vi "ID Finder.vi"(6 "cluster":T3 {"data[0]"."payload" format="%x"; "data[0]"."timestamp" format="%<%.7X\n%x>T"; "data[0]"."type" items=["CAN Data"=0, "CAN Remote"=1, "CAN Bus Error"=2, "CAN 2.0 Data"=8, "CAN FD Data"=16, "CAN FD+BRS Data"=24, "J1939 Data"=192, "Delay"=224, "Log Trigger"=225, "Start Trigger"=226]; "data[0]"."identifier" format="%x"; "data[1]"."payload" format="%x"; "data[1]"."timestamp" format="%<%.7X\n%x>T"; "data[1]"."type" items=["CAN Data"=0, "CAN Remote"=1, "CAN Bus Error"=2, "CAN 2.0 Data"=8, "CAN FD Data"=16, "CAN FD+BRS Data"=24, "J1939 Data"=192, "Delay"=224, "Log Trigger"=225, "Start Trigger"=226]; "data[1]"."identifier" format="%x"; "data[2]"."payload" format="%x"; "data[2]"."timestamp" format="%<%.7X\n%x>T"; "data[2]"."type" items=["CAN Data"=0, "CAN Remote"=1, "CAN Bus Error"=2, "CAN 2.0 Data"=8, "CAN FD Data"=16, "CAN FD+BRS Data"=24, "J1939 Data"=192, "Delay"=224, "Log Trigger"=225, "Start Trigger"=226]; "data[2]"."identifier" format="%x"; "data[3]"."payload" format="%x"; "data[3]"."timestamp" format="%<%.7X\n%x>T"; "data[3]"."type" items=["CAN Data"=0, "CAN Remote"=1, "CAN Bus Error"=2, "CAN 2.0 Data"=8, "CAN FD Data"=16, "CAN FD+BRS Data"=24, "J1939 Data"=192, "Delay"=224, "Log Trigger"=225, "Start Trigger"=226]; "data[3]"."identifier" format="%x"; "data[4]"."payload" format="%x"; "data[4]"."timestamp" format="%<%.7X\n%x>T"; "data[4]"."type" items=["CAN Data"=0, "CAN Remote"=1, "CAN Bus Error"=2, "CAN 2.0 Data"=8, "CAN FD Data"=16, "CAN FD+BRS Data"=24, "J1939 Data"=192, "Delay"=224, "Log Trigger"=225, "Start Trigger"=226]; "data[4]"."identifier" format="%x"; "data[5]"."payload" format="%x"; "data[5]"."timestamp" format="%<%.7X\n%x>T"; "data[5]"."type" items=["CAN Data"=0, "CAN Remote"=1, "CAN Bus Error"=2, "CAN 2.0 Data"=8, "CAN FD Data"=16, "CAN FD+BRS Data"=24, "J1939 Data"=192, "Delay"=224, "Log Trigger"=225, "Start Trigger"=226]; "data[5]"."identifier" format="%x"; "data[6]"."payload" format="%x"; "data[6]"."timestamp" format="%<%.7X\n%x>T"; "data[6]"."type" items=["CAN Data"=0, "CAN Remote"=1, "CAN Bus Error"=2, "CAN 2.0 Data"=8, "CAN FD Data"=16, "CAN FD+BRS Data"=24, "J1939 Data"=192, "Delay"=224, "Log Trigger"=225, "Start Trigger"=226]; "data[6]"."identifier" format="%x"; "data[7]"."payload" format="%x"; "data[7]"."timestamp" format="%<%.7X\n%x>T"; "data[7]"."type" items=["CAN Data"=0, "CAN Remote"=1, "CAN Bus Error"=2, "CAN 2.0 Data"=8, "CAN FD Data"=16, "CAN FD+BRS Data"=24, "J1939 Data"=192, "Delay"=224, "Log Trigger"=225, "Start Trigger"=226]; "data[7]"."identifier" format="%x"; "data[8]"."payload" format="%x"; "data[8]"."timestamp" format="%<%.7X\n%x>T"; "data[8]"."type" items=["CAN Data"=0, "CAN Remote"=1, "CAN Bus Error"=2, "CAN 2.0 Data"=8, "CAN FD Data"=16, "CAN FD+BRS Data"=24, "J1939 Data"=192, "Delay"=224, "Log Trigger"=225, "Start Trigger"=226]; "data[8]"."identifier" format="%x"}) -> (0 "Data Type":T1 items=["CAN Data"=0, "CAN Remote"=1, "CAN Bus Error"=2, "CAN 2.0 Data"=8, "CAN FD Data"=16, "CAN FD+BRS Data"=24, "J1939 Data"=192, "Delay"=224, "Log Trigger"=225, "Start Trigger"=226], 1 "ID STRING":string, 2 "Payload":u8[](array[numeric]), 3 "Timestamp":timestamp, 4 "Identifier":u32)   [LabVIEW 2022 SP3]
uses:
  <vilib>/xnet/xnet.llb/XNET Frame CAN.ctl
  <vilib>/xnet/xnet.llb/XNET Frame Type CAN.ctl
  C:/Users/k90011005/Desktop/Practicas/C#/String-Hexa/bin/Debug/String-Hexa.dll
  Users/k90011005/Desktop/Practicas/C#/String-Hexa/bin/Debug/String-Hexa.dll
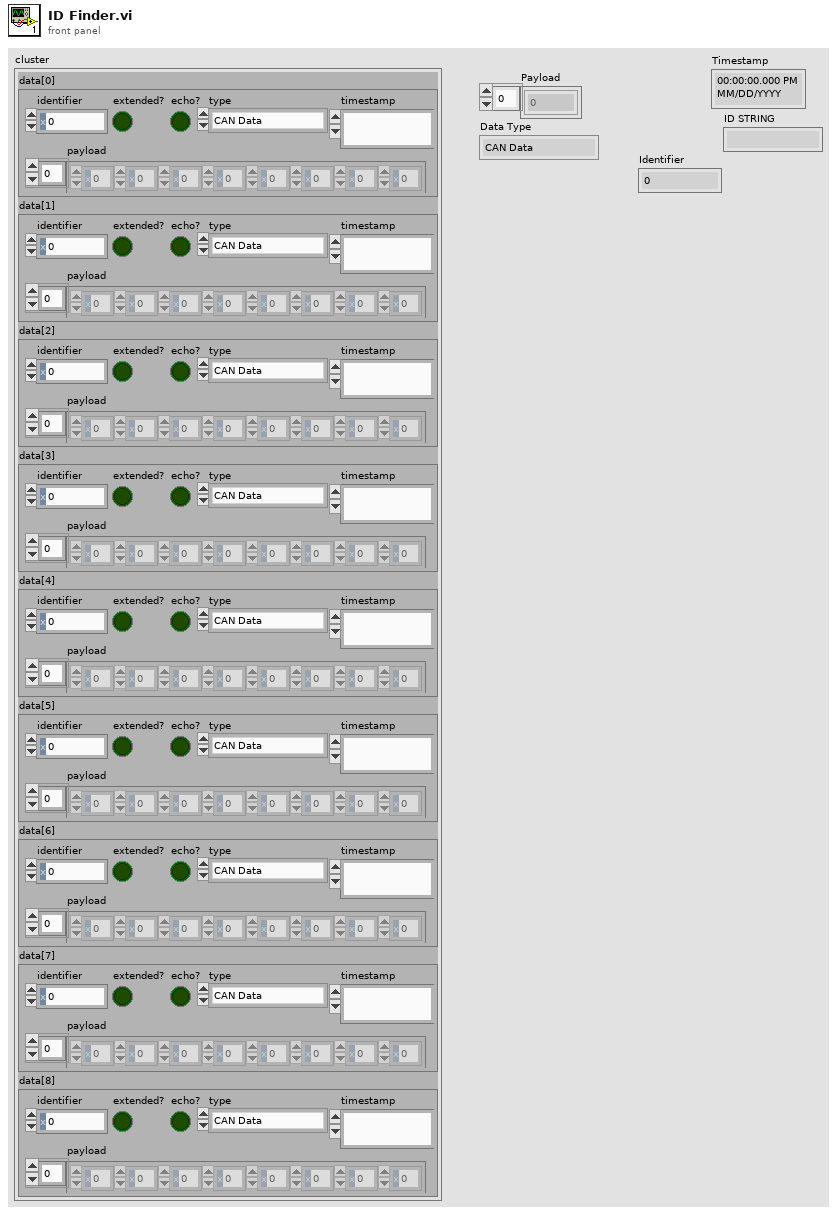
[diagram p1: front panel]
types:
  T1 = typedef "XNET Frame Type CAN.ctl" = u8
  T2 = typedef "XNET Frame CAN.ctl" = cluster{"timestamp":timestamp, "payload":u8[], "identifier":u32, "type":T1, "extended?":bool, "echo?":bool}
  T3 = cluster{"data[0]":T2, "data[1]":T2, "data[2]":T2, "data[3]":T2, "data[4]":T2, "data[5]":T2, "data[6]":T2, "data[7]":T2, "data[8]":T2}
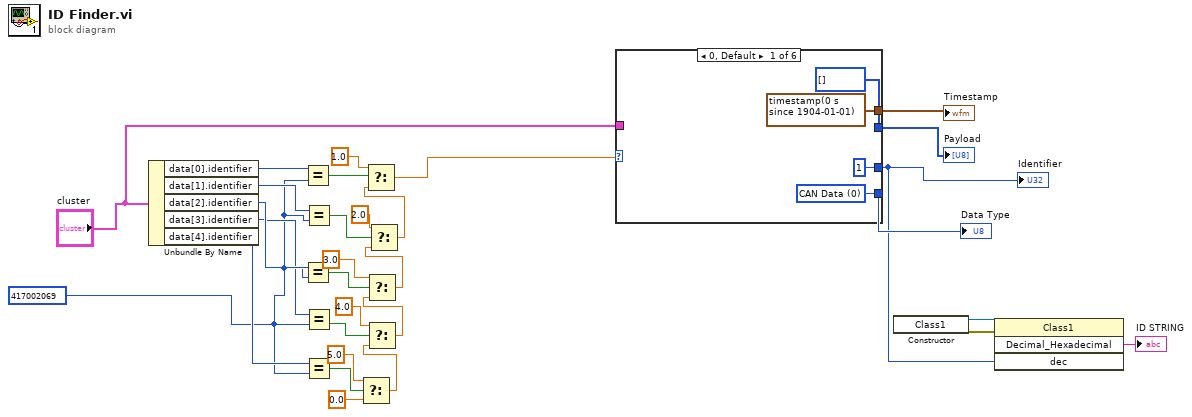
[diagram p0: block diagram]
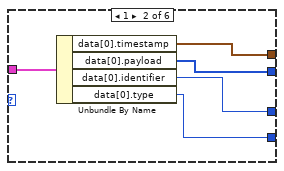
[diagram p2: hidden frame]
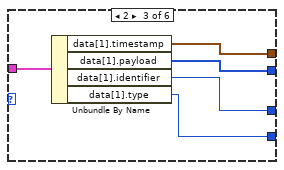
[diagram p3: hidden frame]
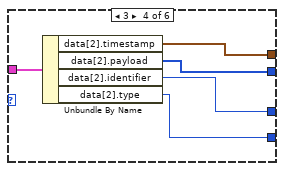
[diagram p4: hidden frame]
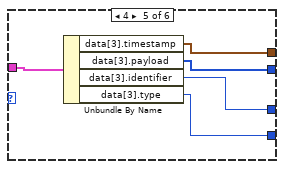
[diagram p5: hidden frame]
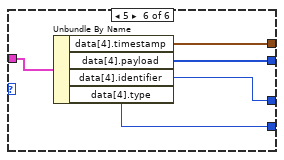
[diagram p6: hidden frame]
diagram:
  w21 = u32 417002069 ("y")
  n1 = Unbundle By Name("cluster") -> ("data[0].identifier"=w30:u32, "data[1].identifier"=w25:u32, "data[2].identifier"=w24:u32, "data[3].identifier"=w23:u32, "data[4].identifier"=w22:u32)
  n2 = Equal?(x=w30, y=w21) -> (x = y?=w29:bool)
  n3 = Equal?(x=w24, y=w21) -> (x = y?=w15:bool)
  n4 = Equal?(x=w25, y=w21) -> (x = y?=w16:bool)
  n5 = Equal?(x=w23, y=w21) -> (x = y?=w14:bool)
  n6 = Equal?(x=w22, y=w21) -> (x = y?=w13:bool)
  n7 = Select(t=5.0, s=w13, f=0.0) -> (s? t:f=w17:dbl)
  n8 = Select(t=4.0, s=w14, f=w17) -> (s? t:f=w18:dbl)
  n9 = Select(t=3.0, s=w15, f=w18) -> (s? t:f=w19:dbl)
  n10 = Select(t=2.0, s=w16, f=w19) -> (s? t:f=w20:dbl)
  n11 = Select(t=1.0, s=w29, f=w20) -> (s? t:f=w27:dbl)
  n12 = case shown="0, Default" w27 {
    tunnel: "cluster" -> [_ w39 w44 w49 w54 w59]
    tunnel: [timestamp(0 s since 1904-01-01) ("timestamp") w38 w43 w48 w53 w58] -> w7
    tunnel: [u8[] [] ("payload") w37 w42 w47 w52 w57] -> w6
    tunnel: [u32 1 ("identifier") w36 w41 w46 w51 w56] -> w2
    tunnel: [w31 w35 w40 w45 w50 w55] -> w5
    frame 0, Default {
      w31 = T1 0 items=["CAN Data"=0, "CAN Remote"=1, "CAN Bus Error"=2, "CAN 2.0 Data"=8, "CAN FD Data"=16, "CAN FD+BRS Data"=24, "J1939 Data"=192, "Delay"=224, "Log Trigger"=225, "Start Trigger"=226] ("type")
    }
    frame 1 {
      n13 = Unbundle By Name(w39) -> ("data[0].timestamp"=w38:timestamp, "data[0].payload"=w37:u8[], "data[0].identifier"=w36:u32, "data[0].type"=w35:T1)
    }
    frame 2 {
      n14 = Unbundle By Name(w44) -> ("data[1].timestamp"=w43:timestamp, "data[1].payload"=w42:u8[], "data[1].identifier"=w41:u32, "data[1].type"=w40:T1)
    }
    frame 3 {
      n15 = Unbundle By Name(w49) -> ("data[2].timestamp"=w48:timestamp, "data[2].payload"=w47:u8[], "data[2].identifier"=w46:u32, "data[2].type"=w45:T1)
    }
    frame 4 {
      n16 = Unbundle By Name(w54) -> ("data[3].timestamp"=w53:timestamp, "data[3].payload"=w52:u8[], "data[3].identifier"=w51:u32, "data[3].type"=w50:T1)
    }
    frame 5 {
      n17 = Unbundle By Name(w59) -> ("data[4].timestamp"=w58:timestamp, "data[4].payload"=w57:u8[], "data[4].identifier"=w56:u32, "data[4].type"=w55:T1)
    }
  }
  "Timestamp" <- w7
  "Payload" <- w6
  "Identifier" <- w2
  "Data Type" <- w5
  n18 = constructor class="Class1"() -> (reference out=w4:refnum<k24>, error out=w3:errorcluster)  [unwired: 3 in, 1 out]
  n19 = invoke class="Class1" method="Decimal_Hexadecimal"(reference=w4, error in=w3, "dec"=w2) -> ("Decimal_Hexadecimal"=→"ID STRING":string)  [unwired: 1 in, 3 out]
